vi "TCP_COMM_ACTV.vi"() -> ()   [LabVIEW 2012]
doc: "接続されたホストと、対話式ダイアログでの会話(TCP接続)を行います。リストにあるマシンと指定されたポートの接続を確立します。接続が確立すると、ユーザによって入力ライン文字列制御器にデータが入力され、Enterキーが押されるまで待機します。Enterキーを押すと入力した文字列がポートに送信され、TCP Communicator - Passive.viは受け取った文字列を表示器に表示します。\n\nActiveとPassive VIの主な違いはActive VIは接続を確立するのに対してPassive VIは接続が確立されるまで待機する点です。\n\n<B>メモ：</B>TCP Communicator - Passive.viが必要です。"
panel:
  in  "Port":u16=7568 caption="ポート"
  in  "Machine":string="localhost" caption="マシン"
  out "Their Response:":string caption="応答："
  in  "stop":bool caption="停止"
  out "You Typed:":string caption="入力した文字列："
  in  "Input Line":string caption="入力文字列"
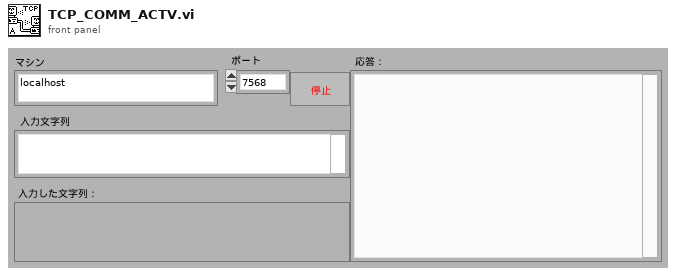
[diagram p1: front panel]
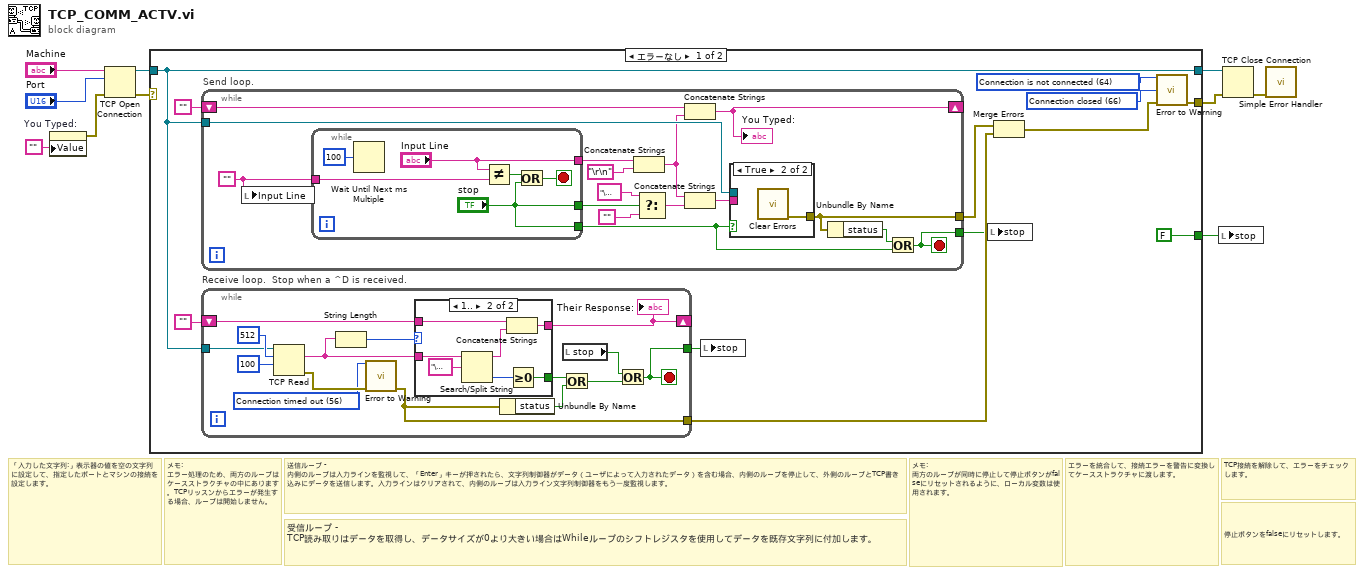
[diagram p0: block diagram]
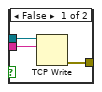
[diagram p2: hidden frame]
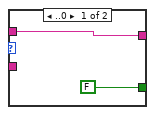
[diagram p3: hidden frame]
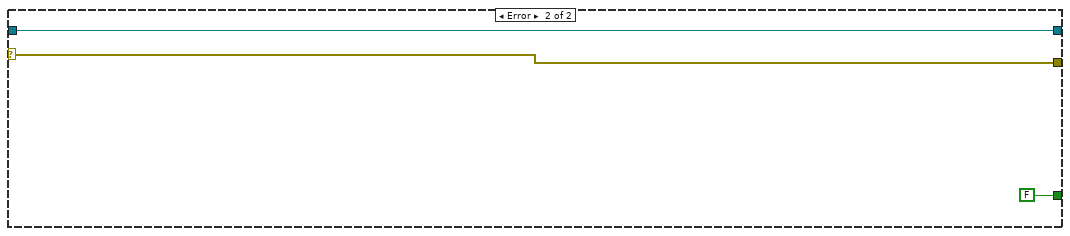
[diagram p4: hidden frame]
diagram:
  # "「入力した文字列:」表示器の値を空の文字列に設定して、指定したポートとマシンの接続を設定します。"
  # "送信ループ - 内側のループは入力ラインを監視して、「Enter」キーが押されたら、文字列制御器がデータ（ユーザによって入力されたデータ）を含む場合、内側のループを停止して、外側のループとTCP書き込みにデータを送信します。入力ラインはクリアされて、内側のループは入力ライン文字列制御器をもう一度監視します。"
  # "受信ループ - TCP読み取りはデータを取得し、データサイズが0より大きい場合はWhileループのシフトレジスタを使用してデータを既存文字列に付加します。"
  # "メモ: 両方のループが同時に停止して停止ボタンがfalseにリセットされるように、ローカル変数は使用されます。"
  # "エラーを統合して、接続エラーを警告に変換してケースストラクチャに渡します。"
  # "メモ:  エラー処理のため、両方のループはケースストラクチャの中にあります。TCPリッスンからエラーが発生する場合、ループは開始しません。"
  # "TCP接続を解除して、エラーをチェックします。"
  # "停止ボタンをfalseにリセットします。"
  n1 = property on="You Typed:" class="Str"("Value"="") -> (error out=w5:errorcluster)  [unwired: 2 in, 1 out]
  n2 = TCP Open Connection(address="Machine", remote port or service name="Port", error in (no error)=w5) -> (connection ID=w7:refnum<k5>, error out=w8:errorcluster)  [unwired: 2 in]
  n3 = case shown="エラーなし" w8 {
    selector: w8 -> [_ w74]
    tunnel: [w14 w74] -> w3
    tunnel: w7 -> [w20 w75]
    tunnel: [w20 w75] -> w4
    tunnel: [FALSE FALSE] -> w1
    frame No Error {
      w15 = 66 items=["No Error", "Argument Error", "Memory Full", "Out of Zone", "End of File", "File Already Open", "Generic File IO Error", "File Not Found", "File Permission Error", "Disk Full", "Duplicate Path", "Too Many Files Open", "Not Enabled", "Resource File Not Found", "Cannot Add Resource", "Resource Not Found", "Image Not Found", "Image Memory Error", "Pen Does Not Exist", "Config Bad Type", "Config Token Not Found", "Config Parse Error", "Config Memory Error", "Bad External Code Format", "Bad External Code Offset", "External Code Not Present", "Null Window", "Destroy Window Mixup", "Null Menu", "Print Aborted", "Bad Print Record", "Print Driver Error", "Windows Error During Print", "Memory Error During Print", "Print Dialog Error", "Generic Print Error", "Invalid Device Refnum", "Device Not Found", "Device Parameter Error", "Device Unit Error", "Can't Open Device", "Device Call Aborted", "Generic Error", "Cancelled By User", "Object ID Too Low", "Object ID Too High", "Object Not In Heap", "Unknown Heap", "Bad DefProc ID", "DefProc Not In Table", "Message Out Of Range", "Null Method", "Unknown Message", "Manager Call Not Supported", "Bad address", "Connection In progress", "Connection timed out", "Connection is already in progress", "Network attribute not supported", "Network error", "Address in use", "System out of memory", "Connection aborted", "Connection refused", "Connection is not connected", "Connection is already connected", "Connection closed", "Initialize error (interapplication manager)", "Bad occurrence", "Wait on unbound occurrence handler", "Occurrence queue overflow", "Bad path", "Semaphore not signaled", "Unrecognized type (interapplication manager)"] ("3rd Error to Convert")
      w16 = 64 items=["No Error", "Argument Error", "Memory Full", "Out of Zone", "End of File", "File Already Open", "Generic File IO Error", "File Not Found", "File Permission Error", "Disk Full", "Duplicate Path", "Too Many Files Open", "Not Enabled", "Resource File Not Found", "Cannot Add Resource", "Resource Not Found", "Image Not Found", "Image Memory Error", "Pen Does Not Exist", "Config Bad Type", "Config Token Not Found", "Config Parse Error", "Config Memory Error", "Bad External Code Format", "Bad External Code Offset", "External Code Not Present", "Null Window", "Destroy Window Mixup", "Null Menu", "Print Aborted", "Bad Print Record", "Print Driver Error", "Windows Error During Print", "Memory Error During Print", "Print Dialog Error", "Generic Print Error", "Invalid Device Refnum", "Device Not Found", "Device Parameter Error", "Device Unit Error", "Can't Open Device", "Device Call Aborted", "Generic Error", "Cancelled By User", "Object ID Too Low", "Object ID Too High", "Object Not In Heap", "Unknown Heap", "Bad DefProc ID", "DefProc Not In Table", "Message Out Of Range", "Null Method", "Unknown Message", "Manager Call Not Supported", "Bad address", "Connection In progress", "Connection timed out", "Connection is already in progress", "Network attribute not supported", "Network error", "Address in use", "System out of memory", "Connection aborted", "Connection refused", "Connection is not connected", "Connection is already connected", "Connection closed", "Initialize error (interapplication manager)", "Bad occurrence", "Wait on unbound occurrence handler", "Occurrence queue overflow", "Bad path", "Semaphore not signaled", "Unrecognized type (interapplication manager)"] ("1st Error to Convert")
      n4 = while "Send loop." {
        tunnel: w20 -> [w35]
        tunnel: [w37] -> w13
        tunnel: [w26] -> w18
        shift-left: "" -> [w38]
        shift-right: [w36] -> _
        stop <- w37 stop-if-true
        w24 = ""
        n5 = local write "Input Line"(w24) -> ()
        n6 = while {
          tunnel: ["stop"] -> w31
          tunnel: ["stop"] -> w23
          tunnel: ["Input Line"] -> w32
          tunnel: w24 -> [w40]
          stop <- w42 stop-if-true
          n7 = Wait Until Next ms Multiple(millisecond multiple=u32 100) -> ()  [unwired: 1 out]
          n8 = Not Equal?(x="Input Line", y=w40) -> (x != y?=w43:bool)
          n9 = Or(x=w43, y="stop") -> (x .or. y?=w42:bool)
        }
        n10 = Concatenate Strings(w32, "\r\n") -> (w28:string)
        n11 = Select(t="\u0004", s=w31, f="") -> (s? t:f=w33:string)
        n12 = Concatenate Strings(w38, w28) -> (w36:string)
        "You Typed:" <- w36
        n13 = Concatenate Strings(w28, w33) -> (w27:string)
        n14 = case shown="TRUE" w23 {
          tunnel: w27 -> [w47 _]
          tunnel: [w46 w48] -> w26
          tunnel: w35 -> [w45 _]
          frame False {
            n15 = TCP Write(connection ID=w45, data in=w47) -> (error out=w46:errorcluster)  [unwired: 2 in, 2 out]
          }
          frame True {
            n16 = call <vilib>:"Clear Errors.vi"() -> ("error out"=w48:errorcluster)  [unwired: 7 in]
          }
        }
        n17 = Unbundle By Name(w26) -> ("status"=w25:bool)
        n18 = Or(x=w25, y=w23) -> (x .or. y?=w37:bool)
      }
      n19 = while "Receive loop.  Stop when a ^D is received." {
        shift-left: "" -> [w60]
        shift-right: [w59] -> _
        tunnel: [w53] -> w19
        tunnel: w20 -> [w61]
        tunnel: [w49] -> w12
        stop <- w49 stop-if-true
        w54 = 56 items=["No Error", "Argument Error", "Memory Full", "Out of Zone", "End of File", "File Already Open", "Generic File IO Error", "File Not Found", "File Permission Error", "Disk Full", "Duplicate Path", "Too Many Files Open", "Not Enabled", "Resource File Not Found", "Cannot Add Resource", "Resource Not Found", "Image Not Found", "Image Memory Error", "Pen Does Not Exist", "Config Bad Type", "Config Token Not Found", "Config Parse Error", "Config Memory Error", "Bad External Code Format", "Bad External Code Offset", "External Code Not Present", "Null Window", "Destroy Window Mixup", "Null Menu", "Print Aborted", "Bad Print Record", "Print Driver Error", "Windows Error During Print", "Memory Error During Print", "Print Dialog Error", "Generic Print Error", "Invalid Device Refnum", "Device Not Found", "Device Parameter Error", "Device Unit Error", "Can't Open Device", "Device Call Aborted", "Generic Error", "Cancelled By User", "Object ID Too Low", "Object ID Too High", "Object Not In Heap", "Unknown Heap", "Bad DefProc ID", "DefProc Not In Table", "Message Out Of Range", "Null Method", "Unknown Message", "Manager Call Not Supported", "Bad address", "Connection In progress", "Connection timed out", "Connection is already in progress", "Network attribute not supported", "Network error", "Address in use", "System out of memory", "Connection aborted", "Connection refused", "Connection is not connected", "Connection is already connected", "Connection closed", "Initialize error (interapplication manager)", "Bad occurrence", "Wait on unbound occurrence handler", "Occurrence queue overflow", "Bad path", "Semaphore not signaled", "Unrecognized type (interapplication manager)"] ("1st Error to Convert")
        n20 = TCP Read(connection ID=w61, bytes to read=512, 9:100) -> (data out=w58:string, error out=w55:errorcluster)  [unwired: 2 in, 1 out]
        n21 = String Length(string=w58) -> (length=w63:i32)
        n22 = call <vilib>:"Error to Warning.vi"("1st Error to Convert"=w54, "error in"=w55) -> ("warning out"=w53:errorcluster)  [unwired: 13 in]
        n23 = case shown="1.." w63 {
          tunnel: w58 -> [_ w69]
          tunnel: w60 -> [w65 w72]
          tunnel: [w65 w71] -> w59
          tunnel: [FALSE w66] -> w57
          frame ..0 {
          }
          frame 1.. {
            n24 = Search/Split String(string=w69, search string/char (-)="\u0004") -> (substring before match=w68:string, offset of match=w67:i32)  [unwired: 1 in, 1 out]
            n25 = Concatenate Strings(w72, w68) -> (w71:string)
            n26 = Greater Or Equal To 0?(x=w67) -> (x >= 0?=w66:bool)
          }
        }
        "Their Response:" <- w59
        n27 = Unbundle By Name(w53) -> ("status"=w52:bool)
        n28 = Or(x=w57, y=w52) -> (x .or. y?=w50:bool)
        n29 = local read "stop"() -> (w51:bool)
        n30 = Or(x=w51, y=w50) -> (x .or. y?=w49:bool)
      }
      n31 = local write "stop"(w12) -> ()
      n32 = local write "stop"(w13) -> ()
      n33 = Merge Errors(w18, w19) -> (w17:errorcluster)
      n34 = call <vilib>:"Error to Warning.vi"("1st Error to Convert"=w16, "3rd Error to Convert"=w15, "error in"=w17) -> ("warning out"=w14:errorcluster)  [unwired: 12 in]
    }
    frame Error {
    }
  }
  n35 = local write "stop"(w1) -> ()
  n36 = TCP Close Connection(connection ID=w4, error in (no error)=w3) -> (error out=w2:errorcluster)  [unwired: 1 in, 1 out]
  n37 = call <vilib>:"Simple Error Handler.vi"("error in (no error)"=w2) -> ()  [unwired: 4 in, 5 out]
